vi "ListTable.vi"(7 "Jsonconfig":string, 8 "error in (no error)":errorcluster, 11 "table":string="TEMATY.uruchomienie_tematy_do_uruchomienia") -> (0 "error out":errorcluster, 3 "data":string[][](array[string]))   [LabVIEW 2015]
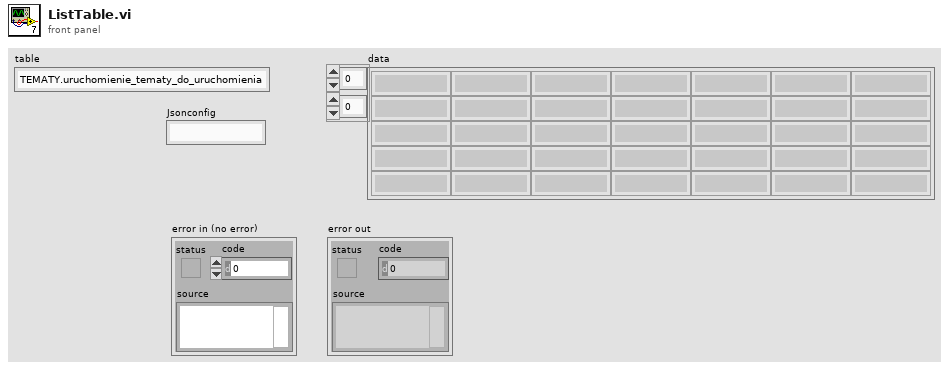
[diagram p1: front panel]
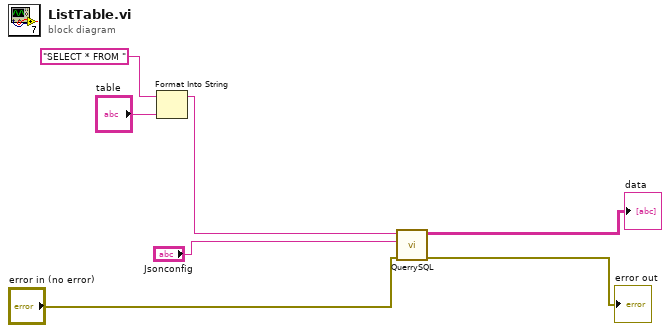
[diagram p0: block diagram]
diagram:
  n1 = Format Into String(initial string="SELECT * FROM ", "table") -> (resulting string=w2:string)  [unwired: 2 in, 1 out]
  n2 = call "QuerrySQL.vi"("error in (no error)"="error in (no error)", "Jsonconfig"="Jsonconfig", "String"=w2) -> ("error out"=→"error out":errorcluster, "Array"=→"data":string[][])  [unwired: 7 in]
